vi "Global var.vi"() -> ()   [LabVIEW 2020]
panel:
  out "ISOBAT-":bool
  out "ISOBAT+":bool
  in  "ODBC":string
  out "RunDCIR":bool
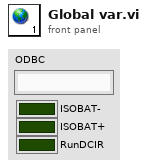
[diagram p1: front panel]
diagram:
